vi "Get Configuration Transfer Filenames.vi"(8 "error in (no error)":errorcluster, 11 "Job Folder":path) -> (0 "error out":errorcluster, 1 "Transfer Files":string[](array[string]), 2 "Job Files":string[](array[string]), 3 "Job Folder out":path)   [LabVIEW 2015]
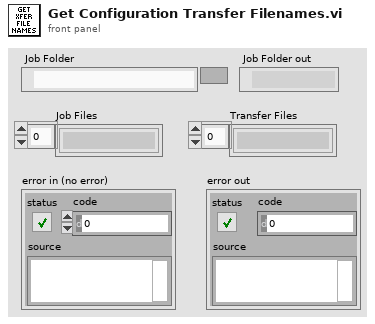
[diagram p1: front panel]
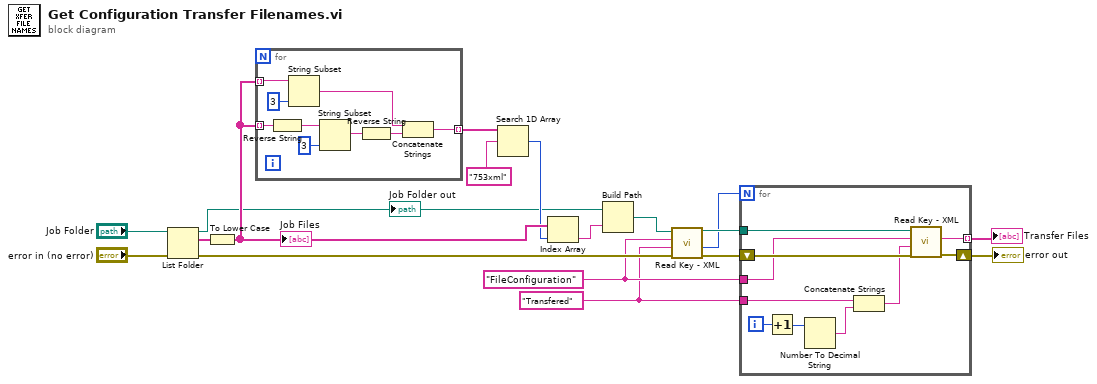
[diagram p0: block diagram]
diagram:
  w4 = "Transfered" ("Section")
  w5 = "FileConfiguration" ("Section")
  n1 = List Folder(path="Job Folder", error in="error in (no error)") -> (path out=w7:path, filenames=w18:string[], error out=w11:errorcluster)  [unwired: 2 in, 1 out]
  "Job Folder out" <- w7
  n2 = To Lower Case(string=w18) -> (all lower case string=w10:string[])
  "Job Files" <- w10
  n3 = for {
    tunnel: w10 -> [w27] mode=indexing
    tunnel: w10 -> [w25] mode=indexing
    tunnel: [w19] -> w15 mode=indexing
    n4 = Reverse String(1:w25) -> (0:w23:string)
    n5 = String Subset(string=w27, length (rest)=3 ("length (rest)")) -> (substring=w20:string)  [unwired: 1 in]
    n6 = String Subset(string=w23, length (rest)=3 ("length (rest)")) -> (substring=w22:string)  [unwired: 1 in]
    n7 = Reverse String(1:w22) -> (0:w21:string)
    n8 = Concatenate Strings(w20, w21) -> (w19:string)
  }
  n9 = Search 1D Array(1D array=w15, element="753xml") -> (index of element=w9:i32)  [unwired: 1 in]
  n10 = Index Array(array=w10, index=w9) -> (element=w8:string)
  n11 = Build Path(base path=w7, name or relative path=w8) -> (appended path=w6:path)
  n12 = call "Read Key - XML.vi"("error in (no error)"=w11, "Key"=w4, "Section"=w5, "XML file"=w6) -> ("error out"=w13:errorcluster, "Value Number"=w1:i32, "XML file out"=w12:path)  [unwired: 4 in, 1 out]
  n13 = for {
    N: w1 -> [_]
    tunnel: w12 -> [w36]
    shift-right: [w29] -> w2
    shift-left: w13 -> [w37]
    tunnel: w5 -> [w35]
    tunnel: w4 -> [w32]
    tunnel: [w28] -> w3 mode=indexing
    i -> [w34]
    n14 = Increment(x=w34) -> (x+1=w33:i32)
    n15 = Number To Decimal String(number=w33) -> (decimal integer string=w31:string)  [unwired: 1 in]
    n16 = Concatenate Strings(w32, w31) -> (w30:string)
    n17 = call "Read Key - XML.vi"("error in (no error)"=w37, "Key"=w30, "Section"=w35, "XML file"=w36) -> ("error out"=w29:errorcluster, "Value String"=w28:string)  [unwired: 4 in, 2 out]
  }
  "error out" <- w2
  "Transfer Files" <- w3
